vi "Identify Measurement Channel Edits.vi"(0 "Queue Ref":refnum<queue>, 1 "Coords":T1, 11 "error in (no error)":errorcluster) -> (6 "Discard?":bool, 15 "error out":errorcluster)   [LabVIEW 2020, in "Plugin.lvlib" / "Plugin_UI.lvclass"]
doc: "Capture the action to be taken for Edits in Input Channel Settings table."
uses:
  Plugin_UI.lvclass
  <vilib>/Utility/miscctls.llb/LVRowAndColumnTypeDef.ctl
  builds/Libraries/Shared GUI Library.lvlibp/Shared GUI Library/Queue Driver/Typedefs/Data.ctl
  builds/Libraries/Shared GUI Library.lvlibp/Shared GUI Library/Queue Driver/Typedefs/Operation.ctl
  builds/Libraries/Shared GUI Library.lvlibp/Shared GUI Library/Queue Driver/Queue Driver.lvlib
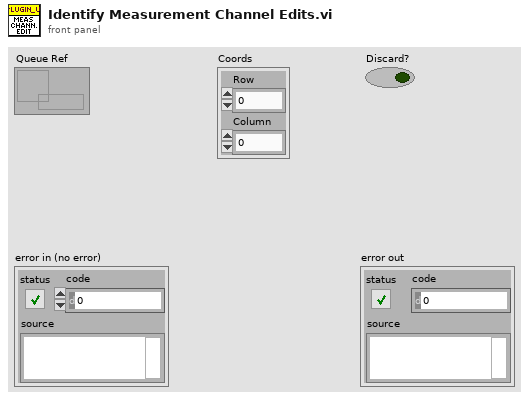
[diagram p1: front panel]
types:
  T1 = typedef "LVRowAndColumnTypeDef.ctl" = cluster{"Row":i32, "Column":i32}
  T2 = typedef "Shared GUI Library.lvlibp/Queue Driver.lvlib/Operation.ctl" = enum16{"Create", "Enqueue without Data", "Enstack without Data", "Enqueue N Elements without Data", "Enqueue with Data", "Enstack with Data", "Enqueue N Elements with Data", "Dequeue", "Flush", "Release"}
  T3 = typedef "Shared GUI Library.lvlibp/Queue Driver.lvlib/Data.ctl" = cluster{"State":string, "Data":variant}
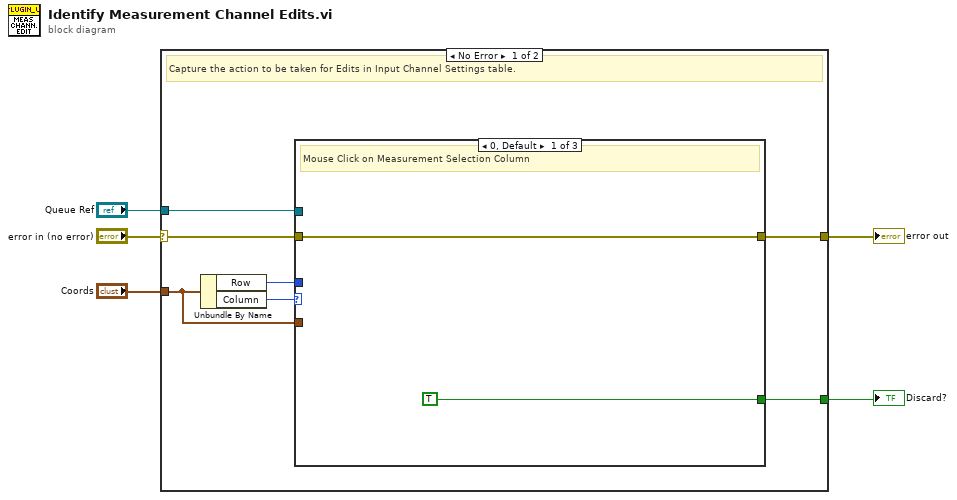
[diagram p0: block diagram]
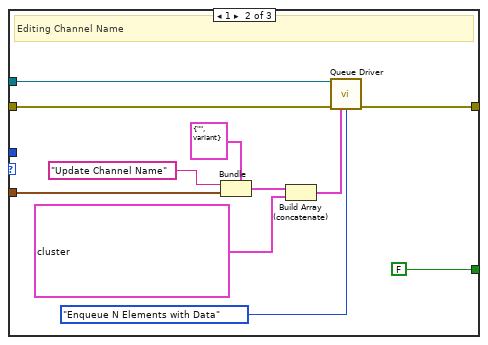
[diagram p2: hidden frame]
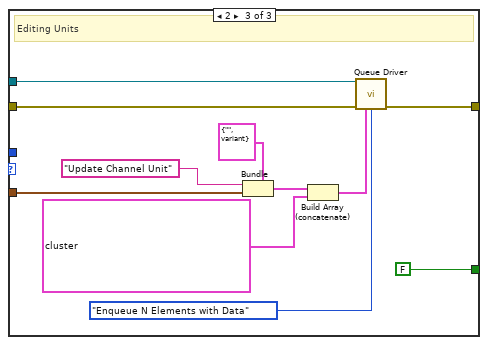
[diagram p3: hidden frame]
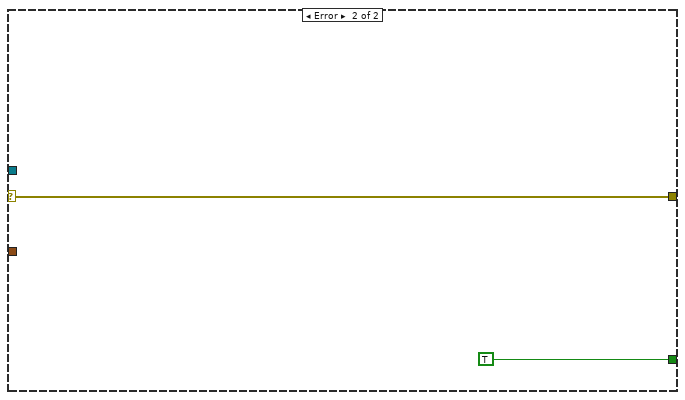
[diagram p4: hidden frame]
diagram:
  n1 = case shown="No Error" "error in (no error)" {
    selector: "error in (no error)" -> [w9 w38]
    tunnel: [w12 TRUE] -> w5
    tunnel: "Coords" -> [w11 _]
    tunnel: [w7 w38] -> w3
    tunnel: "Queue Ref" -> [w6 _]
    frame No Error {
      # "Capture the action to be taken for Edits in Input Channel Settings table."
      n2 = Unbundle By Name(w11) -> ("Row"=w8:i32, "Column"=w10:i32)
      n3 = case shown="0, Default" w10 {
        tunnel: [w13 w18 w28] -> w7
        tunnel: w9 -> [w13 w19 w29]
        tunnel: [TRUE FALSE FALSE] -> w12
        tunnel: w11 -> [_ w20 w31]
        tunnel: w8 -> [_ _ _]
        tunnel: w6 -> [_ w15 w30]
        frame 0, Default {
          # "Mouse Click on Measurement Selection Column"
        }
        frame 1 {
          # "Editing Channel Name"
          n4 = Bundle(cluster=T3 {"State"="", "Data"=variant} ("State with Data"), "State"="Update Channel Name", "Data"=w20) -> (w22:T3)
          n5 = Build Array (concatenate)(w22, T3[] [{"State"="Save Runtime Info", "Data"=variant}, {"State"="CheckForUnsavedChanges", "Data"=variant}] ("State with Data[]")) -> (w17:T3[])
          n6 = call "Queue Driver.vi"("Queue In"=w15, "error in (no error)"=w19, "State with Data[]"=w17, "Operation"=Operation."Enqueue N Elements with Data") -> ("error out"=w18:errorcluster)  [unwired: 8 in, 3 out]
        }
        frame 2 {
          # "Editing Units"
          n7 = Bundle(cluster=T3 {"State"="", "Data"=variant} ("State with Data"), "State"="Update Channel Unit", "Data"=w31) -> (w33:T3)
          n8 = Build Array (concatenate)(w33, T3[] [{"State"="Save Runtime Info", "Data"=variant}, {"State"="CheckForUnsavedChanges", "Data"=variant}, {"State"="Update User Interface", "Data"=variant}] ("State with Data[]")) -> (w27:T3[])
          n9 = call "Queue Driver.vi"("Queue In"=w30, "error in (no error)"=w29, "State with Data[]"=w27, "Operation"=Operation."Enqueue N Elements with Data") -> ("error out"=w28:errorcluster)  [unwired: 8 in, 3 out]
        }
      }
    }
    frame Error {
    }
  }
  "Discard?" <- w5
  "error out" <- w3
